vi "irisOpen.vi"   [LabVIEW 2017]
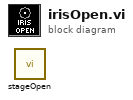
[diagram p0: block diagram]
diagram:
  n1 = call "stageOpen.vi"() -> ()  [unwired: 2 out]
